vi "发送测试命令.vi"(11 "VISA资源名称":refnum<visa-resource-name>) -> (3 "match?":bool)   [LabVIEW 2016, in "DGUS.lvlib" / "DGUS.lvclass"]
uses:
  DGUS.lvclass
  <vilib>/Instr/_visa.llb/VISA Configure Serial Port (Instr).vi
panel:
  out "读取缓冲区":string
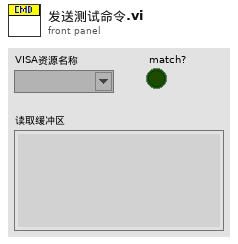
[diagram p1: front panel]
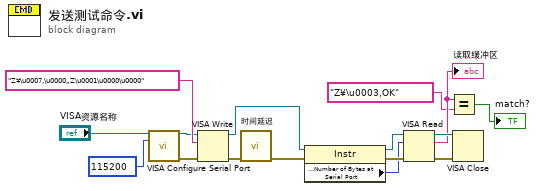
[diagram p0: block diagram]
diagram:
  n1 = call-poly "VISA Configure Serial Port"("VISA resource name"="VISA资源名称", "baud rate (9600)"=u32 115200) -> ("VISA resource name out"=w7:refnum<visa-resource-name>, "error out"=w6:errorcluster)  [unwired: 12 in]
  n2 = VISA Write(VISA resource name=w7, write buffer="Z¥\u0007‚\u0000„Z\u0001\u0000\u0000" ("字符串"), error in (no error)=w6) -> (VISA resource name out=w14:refnum<visa-resource-name>, error out=w15:errorcluster)  [unwired: 1 out]
  n3 = call "时间延迟"("error in (no error)"=w15) -> ("error out"=w13:errorcluster)  [unwired: 10 in]
  n4 = property class="Instr"(reference=w14, error in=w13) -> (reference out=w11:refnum<visa-resource-name>, error out=w12:errorcluster, "Serial Settings:Number of Bytes at Serial Port"=w8:u32)
  n5 = VISA Read(VISA resource name=w11, byte count=w8, error in (no error)=w12) -> (VISA resource name out=w10:refnum<visa-resource-name>, read buffer=w4:string, error out=w9:errorcluster)  [unwired: 1 out]
  "读取缓冲区" <- w4
  n6 = Equal?(x=w4, y="Z¥\u0003‚OK" ("读取缓冲区")) -> (x = y?=→"match?":bool)
  n7 = VISA Close(VISA resource name=w10, error in (no error)=w9) -> ()  [unwired: 1 out]
